vi "Read Outputs to system.vi"(8 "error in":errorcluster, 11 "WaveformAcq runtime in":refnum<class "WaveformAcq runtime.lvclass">) -> (0 "error out":errorcluster, 2 "Outputs to system":T1, 3 "WaveformAcq runtime out":refnum<class "WaveformAcq runtime.lvclass">)   [LabVIEW 2017, in "WaveformAcq runtime.lvclass"]
uses:
  WaveformAcq runtime.lvclass
  configuration/output data indices.ctl
  WaveformAcq runtime.lvclass/WaveformAcq runtime.ctl
  configuration/WaveformAcq configuration.lvclass
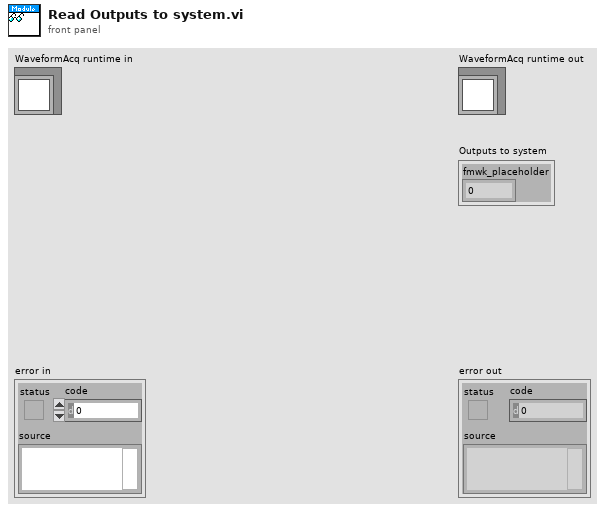
[diagram p1: front panel]
types:
  T1 = typedef "WaveformAcq configuration.lvclass/output data indices.ctl" = cluster{"fmwk_placeholder":i32}
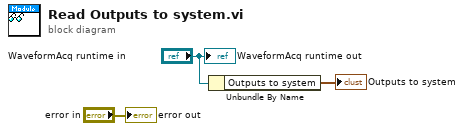
[diagram p0: block diagram]
diagram:
  n1 = Unbundle By Name("WaveformAcq runtime in") -> ("Outputs to system"=→"Outputs to system":T1)
  "error out" <- "error in"
  "WaveformAcq runtime out" <- "WaveformAcq runtime in"
